vi "Measurement UI.vi"() -> ()   [LabVIEW 2025, in "CAN-LIN Raw Bus Capture UI.lvlib"]
uses:
  CAN-LIN Raw Bus Capture UI.lvlib
  Toggle.ctl
  <vilib>/gRPC/LabVIEW gRPC Library/Shared/grpcId.ctl
  <vilib>/Utility/error.llb/whitespace.ctl
  <vilib>/Utility/error.llb/Trim Whitespace One-Sided.vi
  Get Status.vi
  Flush Table.vi
  Create Buffer.vi
  Destroy Table Buffer.vi
  OOB gRPC Client/OOB gRPC Client.lvlib
  <vilib>/gRPC/LabVIEW gRPC Library/grpc-lvsupport-release.lvlib
  Table_Filtering/Table_Filtering.lvlib
panel:
  in  "Tree Data":string[][](array[string])
  in  "Mapping done?":bool
  in  "Table map":map{string, i32}(c390)
  in  "XNET Sessions map":map{u32, refnum<k21>}(c390)
  in  "Tags map":map{string, bool}(c390)
  out "Valid DBC file?":bool
  out "Signals in DBC":i32
  out "Frames in DBC":i32
  in  "Frames Map":map{u32, refnum<k21>}(c390)
  in  "Signals Map":map{u32, refnum<k21>[]}(c390)
  in  "Tree and Table":enum32{"Trace window", "Signal table"}(tab)
  out "Frames":string(tree)
  out "Signals":string[][](table)
  in  "HELP":bool
  out "IsRestarting?":bool
  out "Table Buffer":i32
  out "Error (Logic)":string
  out "Status Message":string
  in  "SAVE FORMAT":u16(ring) items=["TDMS", "CSV"]
  out "Connection":bool
  in  "Clear Trace":bool
  in  "Bus Type":string="CAN"
  in  "Lin Interface":string
  in  "Can Interface":string
  in  "PauseResume":bool
  in  "Path":path
  in  "Save":bool
  in  "Filter":string
  in  "SortByID":bool
  out "Status":string
  in  "SETTINGS":enum32{"CAN", "LIN"}(tab)
  in  "IO Mode":enum32{"CAN", "CAN FD", "CAN FD + BRS"}(ring)
  in  "FD ISO Mode":enum32{"ISO", "Non ISO", "Legacy ISO"}(ring)
  in  "Baudrate":u32=125000
  in  "FD Baudrate":u32=1000000
  in  "Termination CAN":T1
  in  "INTERFACE NAME CAN":refnum<k21>
  in  "DBC path":path
  in  "Termination LIN":T1
  in  "INTERFACE NAME LIN":refnum<k21>
  out "Buffer Size":i32
  out "OOB gRPC Port":i32
  # "CONFIGURATION"
  # "CONTROL"
  # "DBC INFORMATION"
  # "STATUS"
  # "CAN Settings"
  # "LIN Settings"
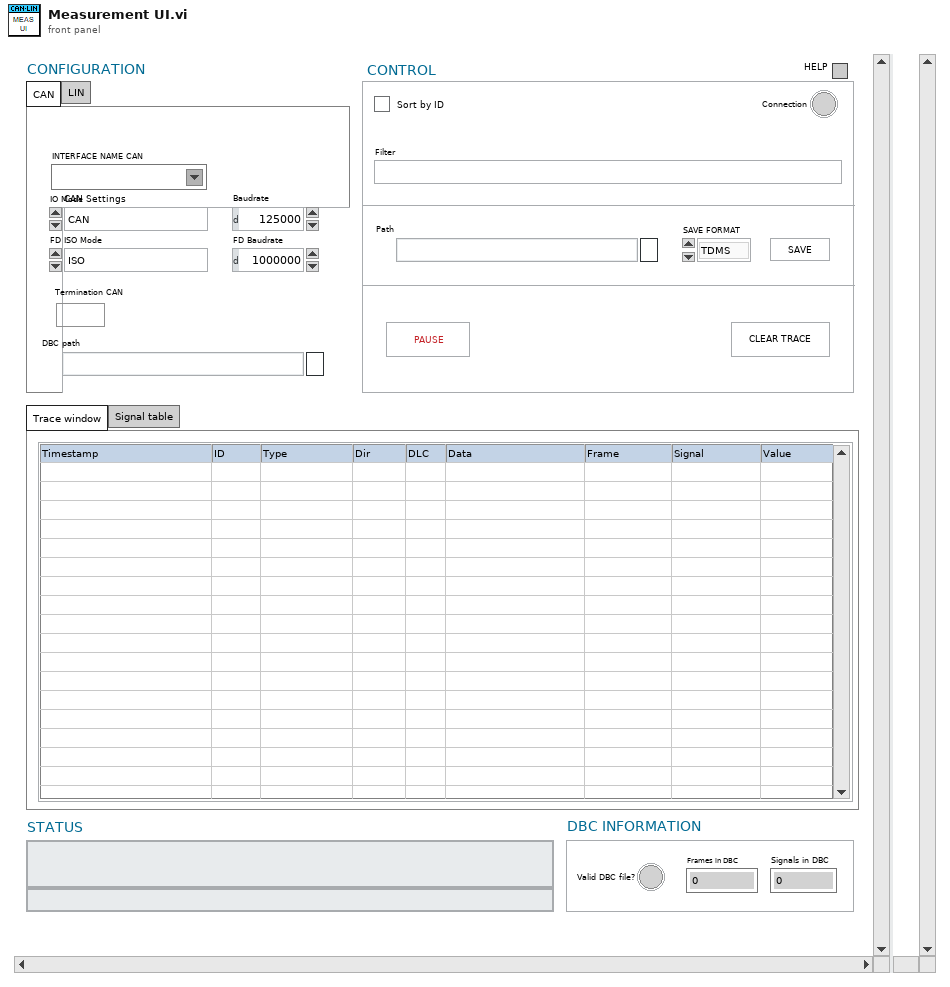
[diagram p1: front panel]
types:
  T1 = typedef "Toggle.ctl" = bool
  T2 = typedef "grpc-lvsupport-release.lvlib/grpcId.ctl" = u64
  T3 = cluster{"Tree Data":refnum<vi>, "Mapping done?":refnum<vi>, "Table map":refnum<vi>, "Tags map":refnum<vi>, "XNET Sessions map":refnum<vi>, "Signals":refnum<vi>, "PauseResume":refnum<vi>, "Clear Trace":refnum<vi>, "Path":refnum<vi>, "SAVE FORMAT":refnum<vi>, "Save":refnum<vi>, "Bus Type":refnum<vi>, "Filter":refnum<vi>, "SortByID":refnum<vi>, "Status Message":refnum<vi>, "Frames":refnum<vi>, "DBC path":refnum<vi>, "Signals Map":refnum<vi>, "Frames Map":refnum<vi>, "Frames in DBC":refnum<vi>, "Signals in DBC":refnum<vi>, "Valid DBC file?":refnum<vi>}
  T4 = typedef "whitespace.ctl" = u16
  T5 = cluster{"FIELD":string, "OPERATOR":string, "VALUE":string}[]
  T6 = enum32{"Page Enabled", "Page Disabled", "Page Disabled & Grayed"}
  T7 = enum8{"Enabled", "Disabled", "Disabled and Grayed Out"}
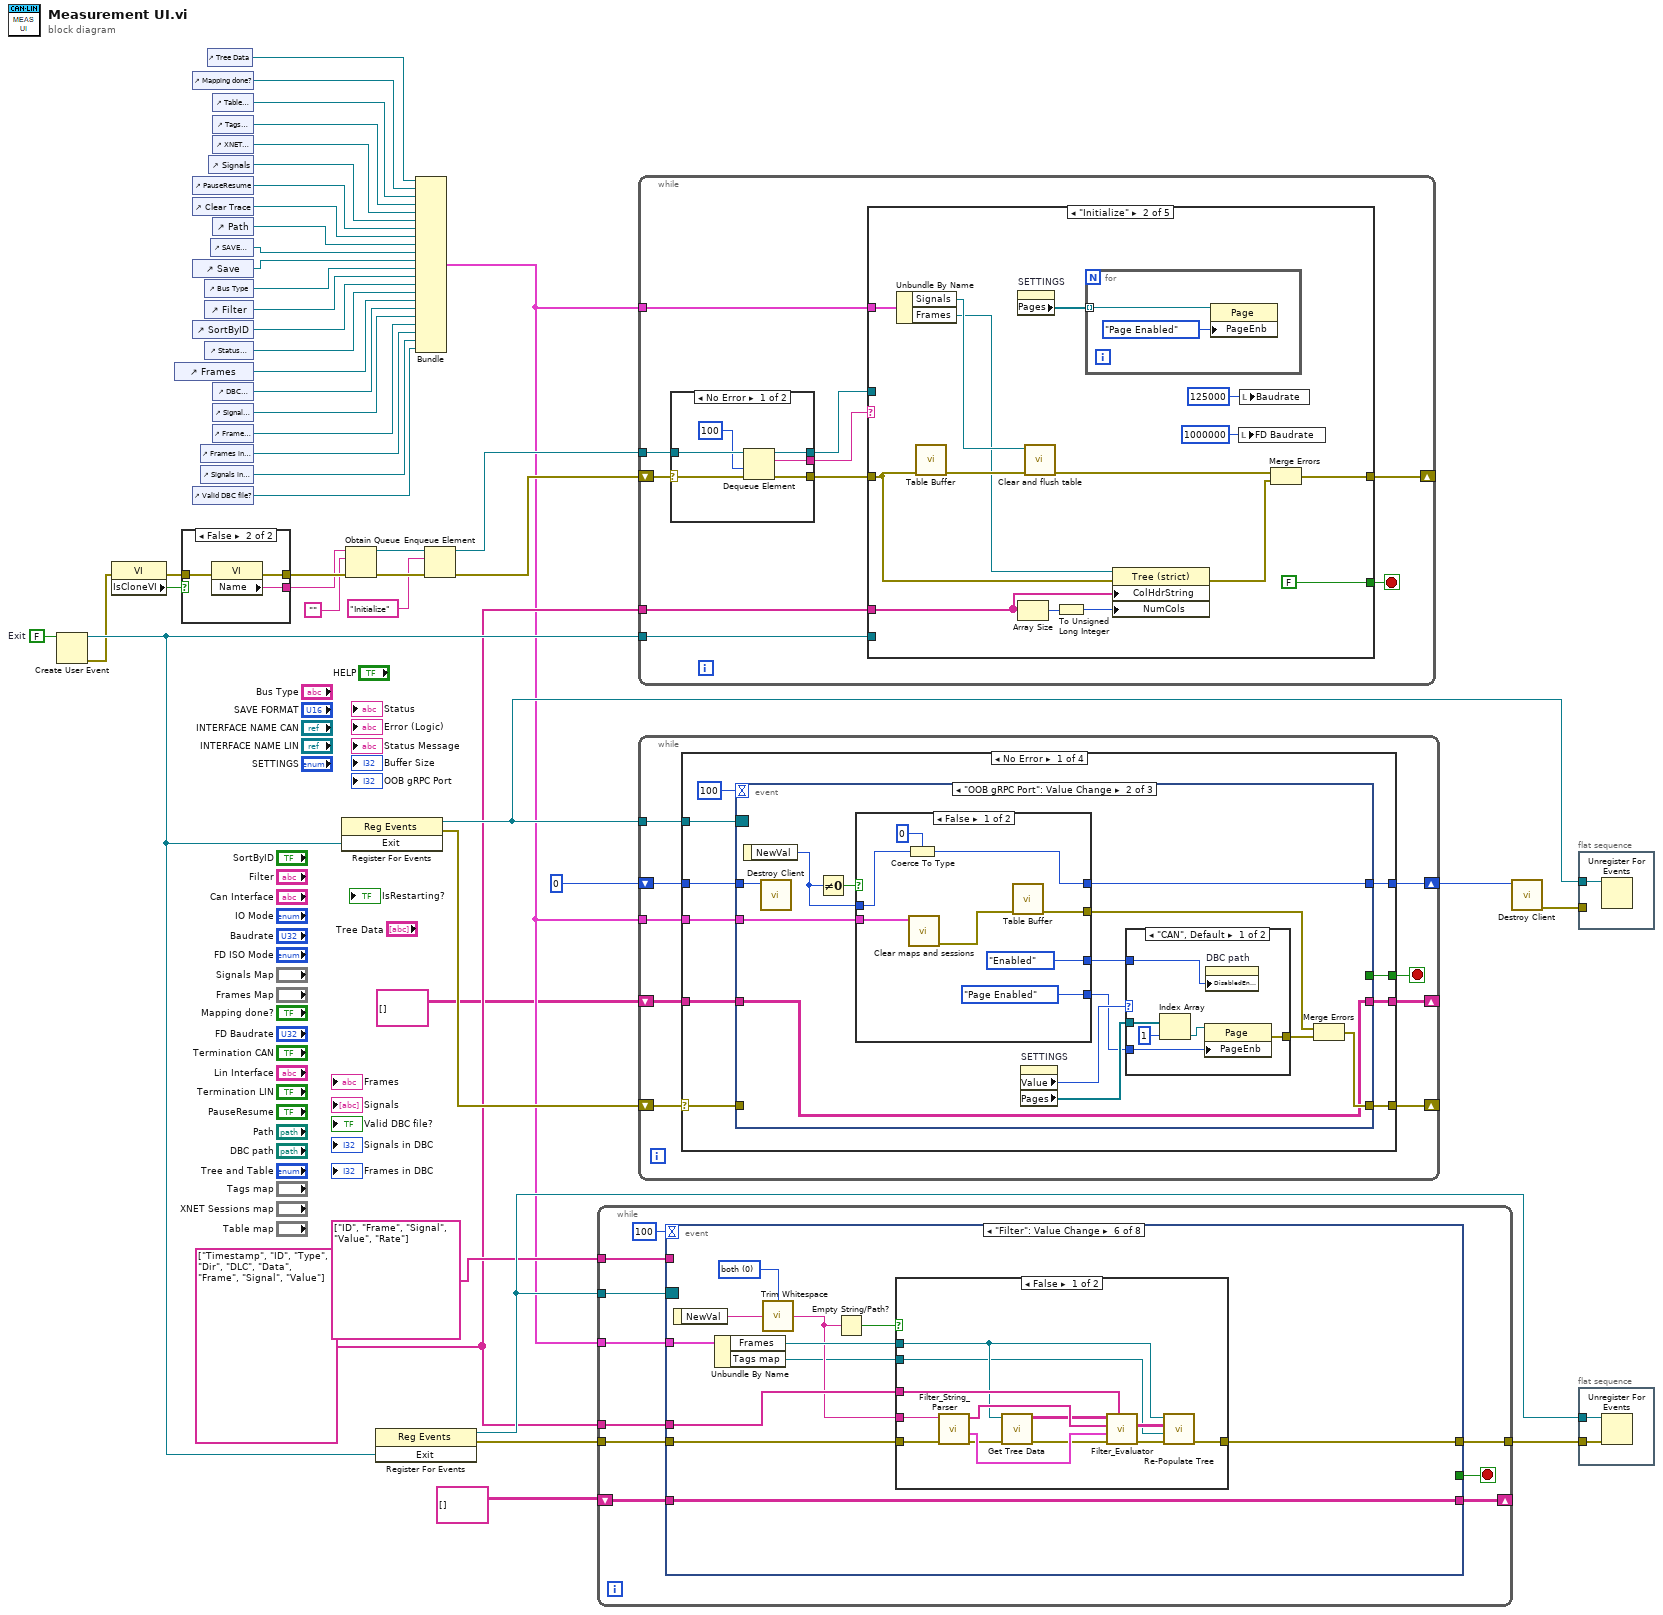
[diagram p0: block diagram]
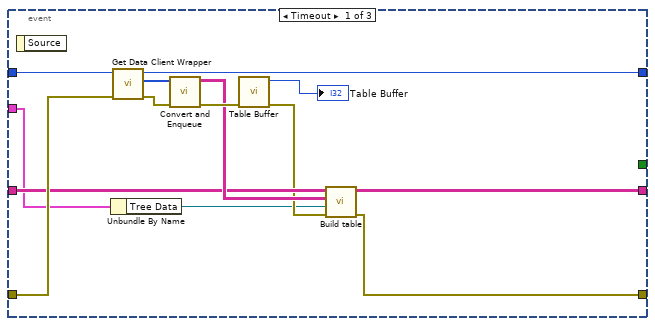
[diagram p2: hidden frame]
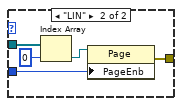
[diagram p3: hidden frame]
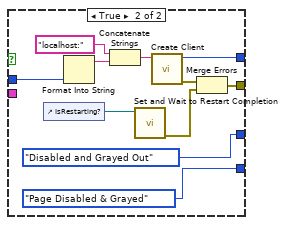
[diagram p4: hidden frame]
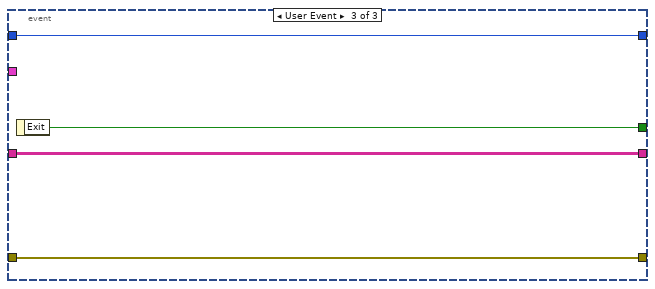
[diagram p5: hidden frame]
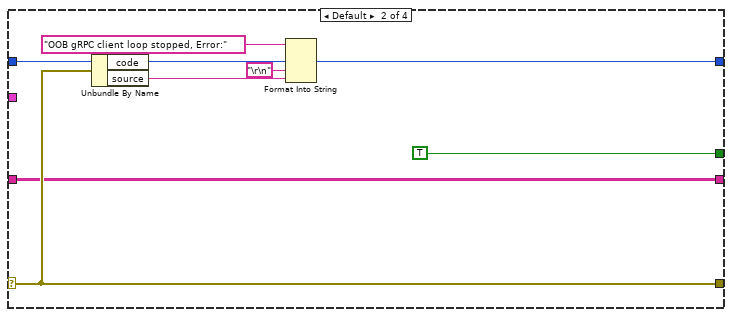
[diagram p6: hidden frame]
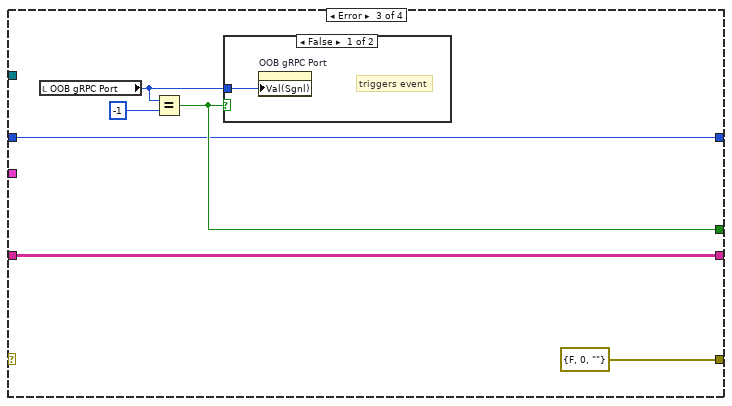
[diagram p7: hidden frame]
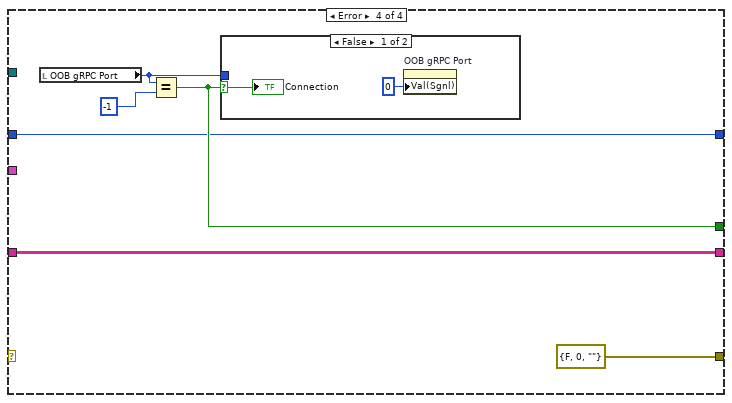
[diagram p9: hidden frame]
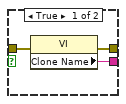
[diagram p11: hidden frame]
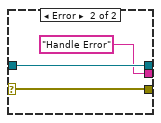
[diagram p12: hidden frame]
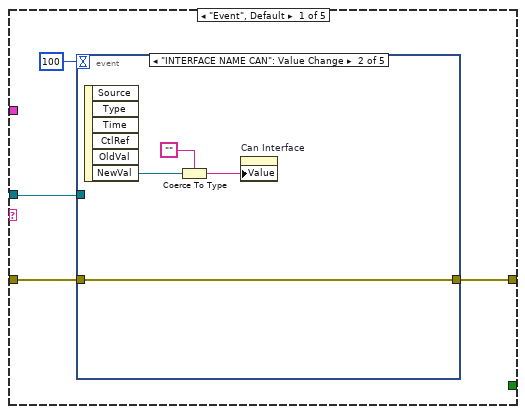
[diagram p13: hidden frame]
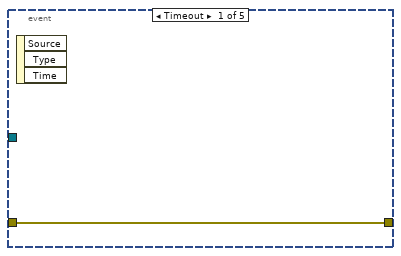
[diagram p14: hidden frame]
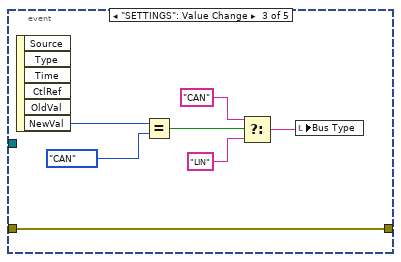
[diagram p15: hidden frame]
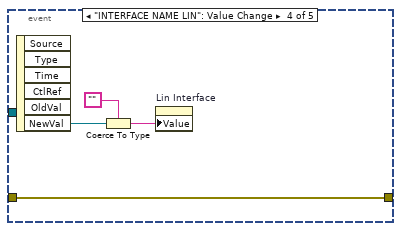
[diagram p16: hidden frame]
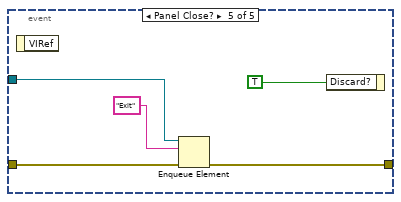
[diagram p17: hidden frame]
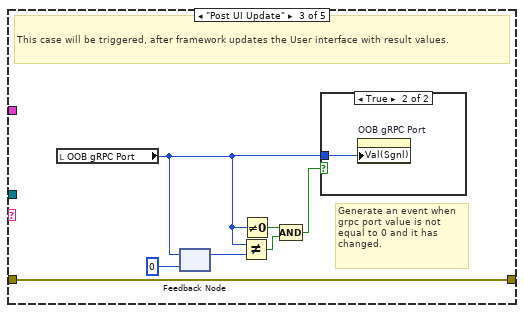
[diagram p18: hidden frame]
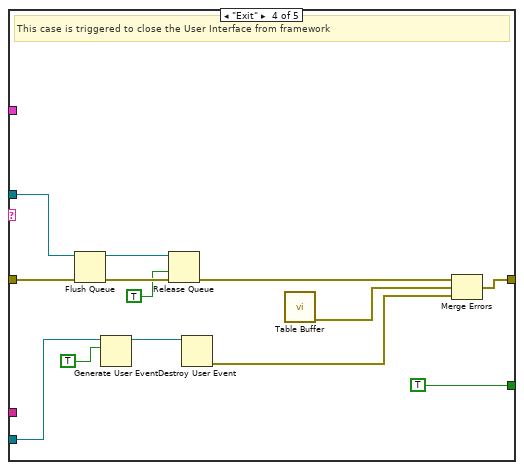
[diagram p20: hidden frame]
diagram:
  w16 = string[] ["Timestamp", "ID", "Type", "Dir", "DLC", "Data", "Frame", "Signal", "Value"] ("Headers")
  w40 = FALSE  # Exit
  n1 = Create User Event(user event datatype=w40) -> (user event=w34:refnum<user-event>, error out=w6:errorcluster)  [unwired: 1 in]
  n2 = property class="VI"(error in=w6) -> (error out=w41:errorcluster, "IsCloneVI"=w42:bool)  [unwired: 1 in, 1 out]
  n3 = control-ref of="Frames"() -> (w20:refnum<vi>)
  n4 = case shown="False" w42 {
    tunnel: [w51 w54] -> w48
    tunnel: [w50 w53] -> w47
    tunnel: w41 -> [w49 w52]
    frame True {
      n5 = property class="VI"(error in=w49) -> (error out=w51:errorcluster, "Clone Name"=w50:string)  [unwired: 1 in, 1 out]
    }
    frame False {
      n6 = property class="VI"(error in=w52) -> (error out=w54:errorcluster, "Name"=w53:string)  [unwired: 1 in, 1 out]
    }
  }
  n7 = control-ref of="Mapping done?"() -> (w4:refnum<vi>)
  n8 = control-ref of="PauseResume"() -> (w24:refnum<vi>)
  n9 = control-ref of="Clear Trace"() -> (w32:refnum<vi>)
  n10 = control-ref of="Save"() -> (w29:refnum<vi>)
  n11 = control-ref of="SortByID"() -> (w27:refnum<vi>)
  n12 = control-ref of="Valid DBC file?"() -> (w12:refnum<vi>)
  n13 = control-ref of="Frames in DBC"() -> (w14:refnum<vi>)
  n14 = control-ref of="Signals in DBC"() -> (w13:refnum<vi>)
  n15 = control-ref of="Bus Type"() -> (w28:refnum<vi>)
  n16 = control-ref of="Filter"() -> (w26:refnum<vi>)
  n17 = control-ref of="Status Message"() -> (w25:refnum<vi>)
  n18 = control-ref of="Tree Data"() -> (w1:refnum<vi>)
  n19 = control-ref of="Signals"() -> (w33:refnum<vi>)
  n20 = control-ref of="SAVE FORMAT"() -> (w30:refnum<vi>)
  n21 = control-ref of="Table map"() -> (w9:refnum<vi>)
  n22 = control-ref of="Tags map"() -> (w11:refnum<vi>)
  n23 = control-ref of="XNET Sessions map"() -> (w10:refnum<vi>)
  n24 = control-ref of="Path"() -> (w31:refnum<vi>)
  n25 = control-ref of="DBC path"() -> (w21:refnum<vi>)
  n26 = control-ref of="Signals Map"() -> (w17:refnum<vi>)
  n27 = control-ref of="Frames Map"() -> (w18:refnum<vi>)
  n28 = register-events(w34) -> (reference out=w36:refnum<event-registration>, error out=w39:errorcluster)  [unwired: 2 in]
  n29 = Obtain Queue(name (unnamed)=w47, element data type="", error in (no error)=w48) -> (queue out=w45:refnum<queue>, error out=w46:errorcluster)  [unwired: 2 in, 1 out]
  n30 = register-events(w34) -> (reference out=w23:refnum<event-registration>, error out=w7:errorcluster)  [unwired: 2 in]
  n31 = Bundle("Tree Data"=w1, "Mapping done?"=w4, "Table map"=w9, "Tags map"=w11, "XNET Sessions map"=w10, "Signals"=w33, "PauseResume"=w24, "Clear Trace"=w32, "Path"=w31, "SAVE FORMAT"=w30, "Save"=w29, "Bus Type"=w28, "Filter"=w26, "SortByID"=w27, "Status Message"=w25, "Frames"=w20, "DBC path"=w21, "Signals Map"=w17, "Frames Map"=w18, "Frames in DBC"=w14, "Signals in DBC"=w13, "Valid DBC file?"=w12) -> (w3:T3)  [unwired: 1 in]
  n32 = Enqueue Element(queue=w45, element="Initialize", error in (no error)=w46) -> (queue out=w15:refnum<queue>, error out=w8:errorcluster)  [unwired: 1 in, 1 out]
  n33 = while {
    tunnel: w7 -> [w64]
    tunnel: [w59] -> w5
    tunnel: w23 -> [w63]
    tunnel: w3 -> [w60]
    shift-right: [w57] -> _
    shift-left: string[][] [] ("Table Data out") -> [w58]
    tunnel: string[] ["ID", "Frame", "Signal", "Value", "Rate"] ("Signal Table Headers") -> [w56]
    tunnel: w16 -> [w55]
    stop <- w62 stop-if-true
    n34 = event shown="[5] \"Filter\": Value Change" {
      selector: w63 -> [_ _ _ _ _ _ _ _]
      dyn-events: _ -> [_ _ _ _ _ _ _ _]
      timeout: 100 -> [_ _ _ _ _ _ _ _]
      tunnel: w64 -> [w82 w94 w113 w130 w154 w165 w186 w188]
      tunnel: [w89 w93 w112 w129 w147 w162 w185 w188] -> w59
      tunnel: [_ _ _ _ _ _ _ w189] -> w62
      tunnel: w60 -> [w80 _ w109 w131 w156 w166 _ _]
      tunnel: w58 -> [w77 w92 w104 w128 w151 w167 w184 w187]
      tunnel: [w91 w92 w105 w128 w151 w167 w184 w187] -> w57
      tunnel: w56 -> [w83 _ _ _ w150 _ _ _]
      tunnel: w55 -> [_ _ _ w126 _ w164 _ _]
      event Timeout {
        n35 = event-data() -> ()  [unwired: 1 in, 1 out]
        n36 = Unbundle By Name(w80) -> ("Signals"=w85:refnum<vi>, "Filter"=w66:refnum<vi>, "SortByID"=w87:refnum<vi>, "Table map"=w78:refnum<vi>, "PauseResume"=w79:refnum<vi>)
        n37 = call "Map the Signals and Frames.vi"("error in"=w82, "References"=w80) -> ("error out"=w81:errorcluster)  [unwired: 9 in]
        n38 = call "PauseResume.vi"("error in"=w81, "PauseResume Ref"=w79) -> ("error out"=w75:errorcluster, "Data"=w84:string[][])  [unwired: 8 in]
        n39 = property class="VI"(error in=w75) -> (error out=w76:errorcluster, "Panel"=w72:refnum<vi>)  [unwired: 1 in, 1 out]
        n40 = property class="Pnl"(reference=w72, error in=w76, "DeferPanUpdts"=TRUE ("Defer Panel Updates")) -> (error out=w74:errorcluster)  [unwired: 1 out]
        n41 = call "Update Trace Tree.vi"("References"=w80, "error in"=w74, "Data IN"=w84) -> ("error out"=w67:errorcluster, "Signals"=w71:string[][])  [unwired: 7 in]
        n42 = call "Update Table.vi"("Table map"=w78, "error in"=w67, "New Data in"=w71, "Table Data in"=w77) -> ("error out"=w68:errorcluster, "Table Data out"=w91:string[][])  [unwired: 6 in]
        n43 = property class="VI"(error in=w68) -> ("Panel"=w69:refnum<vi>)  [unwired: 1 in, 2 out]
        n44 = property class="Pnl"(reference=w69, "DeferPanUpdts"=FALSE ("Defer Panel Updates")) -> (error out=w65:errorcluster)  [unwired: 1 in, 1 out]
        n45 = Empty Array?(array=w71) -> (empty?=w86:bool)
        n46 = call "SortByID.vi"("Headers"=w83, "Trace"=w85, "error in"=w65, "Unsorted Data"=w91, "SortByID"=w87, "Filter"=w66) -> ("error out"=w90:errorcluster, "Table Control"=w88:string[][])  [unwired: 4 in]
        n47 = call "Programatic Scroll.vi"("error in"=w90, "Pause? (F)"=w86, "Table Ref"=w85, "Trace"=w88) -> ("error out"=w89:errorcluster)  [unwired: 7 in]
      }
      event "Clear Trace": Value Change {
        # "Run when restarting or then button is pressed down."
        n48 = event-data() -> ("NewVal"=w95:bool)  [unwired: 1 in]
        n49 = case shown="False" w95 {
          tunnel: w94 -> [w98 w99]
          tunnel: [w96 w99] -> w93
          frame False {
            n50 = property on="IsRestarting?" class="Bool (strict)"(error in=w98, "Val(Sgnl)"=FALSE ("Value (Signaling)")) -> (error out=w96:errorcluster)  [unwired: 1 in, 1 out]
          }
          frame True {
          }
        }
      }
      event "IsRestarting?": Value Change {
        n51 = event-data() -> ("NewVal"=w111:bool)  [unwired: 1 in]
        n52 = Unbundle By Name(w109) -> ("Table map"=w100:refnum<vi>, "Tags map"=w101:refnum<vi>, "Frames"=w102:refnum<vi>, "Status Message"=w106:refnum<vi>, "Signals"=w108:refnum<vi>)
        n53 = Not(x=w111) -> (.not. x?=w110:bool)
        n54 = call "Clear Table.vi"("error in"=w113, "Confirm? (F)"=w110, "Table in"=w108) -> ("error out"=w107:errorcluster, "T button?"=w103:bool)  [unwired: 7 in]
        n55 = case shown="True" w103 {
          tunnel: [w115 w124] -> w112
          tunnel: w107 -> [w115 w122]
          tunnel: w106 -> [_ w121]
          tunnel: [w114 string[][] [] ("Table Data out")] -> w105
          tunnel: w104 -> [w114 _]
          tunnel: w102 -> [_ w118]
          tunnel: w101 -> [_ w117]
          tunnel: w100 -> [_ w116]
          frame False {
          }
          frame True {
            # "Reset Table when necessary"
            n56 = invoke class="Map (strict)" method="Reinit To Default"(reference=w116) -> ()  [unwired: 2 in, 3 out]
            n57 = invoke class="Map (strict)" method="Reinit To Default"(reference=w117) -> ()  [unwired: 2 in, 3 out]
            n58 = property class="Str"(reference=w121, error in=w122, "Value"="") -> (error out=w123:errorcluster)  [unwired: 1 out]
            n59 = property on="IsRestarting?" class="Bool (strict)"(error in=w123, "Value"=FALSE ("IsRestarting?")) -> (error out=w124:errorcluster)  [unwired: 1 in, 1 out]
            n60 = invoke on="Invoke Node" class="Tree (strict)" method="Edit Tree Items.Delete"(reference=w118) -> ()  [unwired: 4 in, 5 out]
          }
        }
      }
      event "Save": Value Change {
        n61 = event-data() -> ("NewVal"=w127:bool)  [unwired: 1 in]
        n62 = case shown="False" w127 {
          tunnel: w131 -> [_ w145]
          tunnel: w130 -> [w132 w141]
          tunnel: [w132 w139] -> w129
          tunnel: w126 -> [_ w137]
          frame True {
          }
          frame False {
            n63 = Unbundle By Name(w145) -> ("DBC path"=w134:refnum<vi>, "Status Message"=w136:refnum<vi>, "Path"=w144:refnum<vi>, "SAVE FORMAT"=w143:refnum<vi>, "Bus Type"=w142:refnum<vi>, "Tree Data"=w133:refnum<vi>, "Frames"=w135:refnum<vi>)
            n64 = call "Save CAN data.vi"("Frames"=w135, "DBC path"=w134, "Tree Data"=w133, "Headers"=w137, "error in"=w141, "Bus Type"=w142, "Format"=w143, "Path"=w144) -> ("error out"=w140:errorcluster, "Status"=w138:string)  [unwired: 2 in]
            n65 = property class="Str"(reference=w136, error in=w140, "Value"=w138) -> (error out=w139:errorcluster)  [unwired: 1 out]
          }
        }
      }
      event "SortByID": Value Change {
        # "This currently only checks the sorting value change,\nmigth need to check the  Filter Value Change too."
        n66 = event-data() -> ()  [unwired: 1 in, 1 out]
        n67 = Unbundle By Name(w156) -> ("Tags map"=w146:refnum<vi>, "Frames"=w149:refnum<vi>, "Signals"=w153:refnum<vi>, "Filter"=w152:refnum<vi>, "SortByID"=w155:refnum<vi>)
        n68 = call "SortByID.vi"("Headers"=w150, "Trace"=w153, "error in"=w154, "Unsorted Data"=w151, "SortByID"=w155, "Filter"=w152) -> ("error out"=w148:errorcluster)  [unwired: 4 in, 1 out]
        n69 = call "Order tree.vi"("Tags map"=w146, "error in"=w148, "TreeControl in"=w149) -> ("error out"=w147:errorcluster)  [unwired: 8 in]
      }
      event "Filter": Value Change {
        w160 = T4 0 items=["both", "start of string", "end of string"] ("location (both)")
        n70 = event-data() -> ("NewVal"=w161:string)  [unwired: 1 in]
        n71 = Unbundle By Name(w166) -> ("Frames"=w163:refnum<vi>, "Tags map"=w157:refnum<vi>)
        n72 = call <vilib>:"Trim Whitespace.vi"("string"=w161, "location (both)"=w160) -> ("trimmed string"=w159:string)
        n73 = Empty String/Path?(string/path=w159) -> (empty?=w158:bool)
        n74 = case shown="False" w158 {
          tunnel: w165 -> [w180 w181]
          tunnel: w164 -> [w177 _]
          tunnel: w163 -> [w171 _]
          tunnel: [w170 w181] -> w162
          tunnel: w159 -> [w169 _]
          tunnel: w157 -> [w168 _]
          frame False {
            n75 = call "Filter_String_Parser.vi"("error in"=w180, "Filter String"=w169) -> ("error constant"=w174:errorcluster, "Comparators"=w179:T5, "Boolean Connectors"=w178:string[])  [unwired: 7 in]
            n76 = call "Get Tree Data.vi"("error in"=w174, "Tree ref"=w171) -> ("error out"=w175:errorcluster, "Array"=w176:string[][])  [unwired: 8 in]
            n77 = call "Filter_Evaluator.vi"("Headers"=w177, "Error"=w175, "Comparators"=w179, "Boolean Connectors"=w178, "Prefiltered Data"=w176) -> ("Error Out"=w172:errorcluster, "Filtered Array"=w173:string[][])  [unwired: 4 in, 1 out]
            n78 = call "Re-Populate Tree.vi"("error in"=w172, "Tags map"=w168, "Data in"=w173, "TreeControl in"=w171) -> ("error out"=w170:errorcluster)  [unwired: 7 in]
          }
          frame True {
          }
        }
      }
      event "HELP": Value Change {
        n79 = event-data() -> ("NewVal"=w183:bool)  [unwired: 1 in]
        n80 = call "Open Help PDF.vi"("error in"=w186, "NewVal"=w183, "Path after documentation"=path "CAN-LIN Raw Bus Capture.pdf") -> ("error out"=w185:errorcluster)  [unwired: 8 in]
      }
      event User Event {
        n81 = event-data() -> ("Exit"=w189:bool)  [unwired: 1 in]
      }
    }
  }
  n82 = while {
    shift-right: [w194] -> _
    shift-left: w8 -> [w199]
    tunnel: w15 -> [w197]
    tunnel: w34 -> [w192]
    tunnel: w3 -> [w191]
    tunnel: w16 -> [w190]
    stop <- w193 stop-if-true
    n83 = case shown="No Error" w199 {
      selector: w199 -> [w205 w208]
      tunnel: [w204 w208] -> w198
      tunnel: w197 -> [w203 w207]
      tunnel: [w202 w207] -> w196
      tunnel: [w201 "Handle Error"] -> w195
      frame No Error {
        n84 = Dequeue Element(queue=w203, timeout in ms (-1)=100, error in (no error)=w205) -> (queue out=w202:refnum<queue>, element=w201:string, error out=w204:errorcluster)  [unwired: 1 out]
      }
      frame Error {
      }
    }
    n85 = case shown="\"Initialize\"" w195 {
      tunnel: w198 -> [w211 w236 w251 w271 w276]
      tunnel: w196 -> [w210 _ _ w269 w275]
      tunnel: [w212 w239 w251 w260 w276] -> w194
      tunnel: [_ FALSE _ TRUE _] -> w193
      tunnel: w192 -> [_ _ _ w263 _]
      tunnel: w191 -> [_ w234 _ _ _]
      tunnel: w190 -> [_ w235 _ _ _]
      frame "Event", Default {
        n86 = event shown="[1] \"INTERFACE NAME CAN\": Value Change" {
          selector: _ -> [_ _ _ _ _]
          dyn-events: _ -> [_ _ _ _ _]
          timeout: 100 -> [_ _ _ _ _]
          tunnel: [w213 w217 w219 w228 w232] -> w212
          tunnel: w211 -> [w213 w217 w219 w228 w233]
          tunnel: w210 -> [_ _ _ _ w231]
          event Timeout {
            n87 = event-data() -> ()  [unwired: 1 in, 3 out]
          }
          event "INTERFACE NAME CAN": Value Change {
            n88 = event-data() -> ("NewVal"=w215:refnum<k21>)  [unwired: 1 in, 5 out]
            n89 = Coerce To Type(0:w215, 1:"") -> (2:w214:string)
            n90 = property on="Can Interface" class="Str"("Value"=w214) -> ()  [unwired: 2 in, 2 out]
          }
          event "SETTINGS": Value Change {
            n91 = event-data() -> ("NewVal"=w224:enum32{"CAN", "LIN"})  [unwired: 1 in, 5 out]
            n92 = Equal?(x=w224, y=enum32{"CAN", "LIN"}."CAN") -> (x = y?=w222:bool)
            n93 = Select(t="CAN", s=w222, f="LIN") -> (s? t:f=w218:string)
            n94 = local write "Bus Type"(w218) -> ()
          }
          event "INTERFACE NAME LIN": Value Change {
            n95 = event-data() -> ("NewVal"=w225:refnum<k21>)  [unwired: 1 in, 5 out]
            n96 = Coerce To Type(0:w225, 1:"") -> (2:w226:string)
            n97 = property on="Lin Interface" class="Str"("Value"=w226) -> ()  [unwired: 2 in, 2 out]
          }
          event Panel Close? {
            n98 = event-data() -> ()  [unwired: 1 in, 1 out]
            n99 = Enqueue Element(queue=w231, element="Exit", error in (no error)=w233) -> (error out=w232:errorcluster)  [unwired: 1 in, 2 out]
            n100 = event-data("Discard?"=TRUE) -> ()  [unwired: 1 in, 1 out]
          }
        }
      }
      frame "Initialize" {
        n101 = Unbundle By Name(w234) -> ("Signals"=w245:refnum<vi>, "Frames"=w240:refnum<vi>)
        n102 = call-poly "Table Buffer.vi"("error in (no error)"=w236) -> ("error out"=w243:errorcluster)  [unwired: 10 in]
        n103 = property on="SETTINGS" class="TabCtl (strict)"() -> ("Pages"=w244:refnum<vi>[])  [unwired: 2 in, 2 out]
        n104 = Array Size(array=w235) -> (size(s)=w241:i32)
        n105 = call "Clear and flush table.vi"("error in"=w243, "Trace"=w245) -> ("error out"=w238:errorcluster)  [unwired: 9 in]
        n106 = To Unsigned Long Integer(number=w241) -> (unsigned 32bit integer=w242:u32)
        n107 = for {
          tunnel: w244 -> [w250] mode=indexing
          n108 = property class="Page"(reference=w250, "PageEnb"=T6."Page Enabled" ("Page Enabled State")) -> ()  [unwired: 1 in, 2 out]
        }
        n109 = property on="Property Node" class="Tree (strict)"(reference=w240, error in=w236, "ColHdrString"=w235, "NumCols"=w242) -> (error out=w237:errorcluster)  [unwired: 1 out]
        n110 = local write "FD Baudrate"(u32 1000000 ("FD Baudrate")) -> ()
        n111 = local write "Baudrate"(u32 125000 ("Baudrate")) -> ()
        n112 = Merge Errors(w238, w237) -> (w239:errorcluster)
      }
      frame "Post UI Update" {
        # "Generate an event when grpc port value is not equal to 0 and it has changed."
        # "This case will be triggered, after framework updates the User interface with result values."
        n113 = local read "OOB gRPC Port"() -> (w254:i32)
        n114 = feedback #1(0 ("OOB gRPC Port")) -> (w253:i32)
        n115 = feedback-in #1(w254) -> ()
        n116 = Not Equal?(x=w254, y=w253) -> (x != y?=w255:bool)
        n117 = Not Equal To 0?(x=w254) -> (x != 0?=w256:bool)
        n118 = Compound Arithmetic op=AND(w256, w255) -> (w252:bool)
        n119 = case shown="True" w252 {
          tunnel: w254 -> [_ w258]
          frame False {
          }
          frame True {
            n120 = property on="OOB gRPC Port" class="DigNum (strict)"("Val(Sgnl)"=w258) -> ()  [unwired: 2 in, 2 out]
          }
        }
      }
      frame "Exit" {
        # "This case is triggered to close the User Interface from framework"
        n121 = Flush Queue(queue=w269, error in (no error)=w271) -> (queue out=w268:refnum<queue>, error out=w267:errorcluster)  [unwired: 1 out]
        n122 = Generate User Event(user event=w263, event data cluster=TRUE ("event data")) -> (user event out=w265:refnum<user-event>)  [unwired: 2 in, 1 out]
        n123 = Release Queue(queue=w268, force destroy? (F)=TRUE, error in (no error)=w267) -> (error out=w259:errorcluster)  [unwired: 2 out]
        n124 = Destroy User Event(user event=w265) -> (error out=w262:errorcluster)  [unwired: 1 in]
        n125 = call-poly "Table Buffer.vi"() -> ("error out"=w261:errorcluster)  [unwired: 11 in]
        n126 = Merge Errors(w259, w261, w262) -> (w260:errorcluster)
      }
      frame "Handle Error" {
        w274 = "UI main loop stopped, Error: %d - %s" ("format string")
        n127 = Unbundle By Name(w276) -> ("code"=w277:i32, "source"=w272:string)
        n128 = case shown="Default" w276 {
          selector: w276 -> [w278 w283]
          tunnel: [w278 w282] -> _
          tunnel: w275 -> [_ w279]
          frame No Error {
          }
          frame Default {
            n129 = call <vilib>:"Clear Errors.vi"("error in (no error)"=w283) -> ("error out"=w281:errorcluster)  [unwired: 5 in, 1 out]
            n130 = Enqueue Element At Opposite End(queue=w279, element="Exit", error in (no error)=w281) -> (error out=w282:errorcluster)  [unwired: 1 in, 2 out]
          }
        }
        n131 = Format Into String(format string=w274, initial string=w274, w277, w272) -> (resulting string=w273:string)  [unwired: 1 in, 1 out]
        n132 = local write "Status Message"(w273) -> ()
      }
    }
  }
  n133 = while {
    tunnel: w36 -> [w289]
    shift-right: [w290] -> _
    shift-left: w39 -> [w292]
    shift-right: [w287] -> w37
    shift-left: T2 0 ("gRPC ID out") -> [w288]
    tunnel: w3 -> [w286]
    shift-right: [w284] -> _
    shift-left: string[][] [] ("Table Data in") -> [w285]
    stop <- w291 stop-if-true
    n134 = case shown="No Error" w292 {
      selector: w292 -> [w300 w365 _ _]
      tunnel: [w297 TRUE w375 w382] -> w291
      tunnel: [w301 w365 errorcluster {"status"=FALSE, "code"=0, "source"=""} ("error IO") errorcluster {"status"=FALSE, "code"=0, "source"=""} ("error IO")] -> w290
      tunnel: w289 -> [w302 _ _ _]
      tunnel: w288 -> [w299 w370 w374 w381]
      tunnel: [w298 w370 w374 w381] -> w287
      tunnel: w286 -> [w295 _ _ _]
      tunnel: w285 -> [w294 w364 w372 w379]
      tunnel: [w293 w364 w372 w379] -> w284
      frame No Error {
        n135 = event shown="[1] \"OOB gRPC Port\": Value Change" {
          selector: w302 -> [_ _ _]
          dyn-events: _ -> [_ _ _]
          timeout: 100 -> [_ _ _]
          tunnel: [w306 w320 w361] -> w301
          tunnel: w300 -> [w310 _ w361]
          tunnel: w299 -> [w311 w329 w362]
          tunnel: [w316 w328 w362] -> w298
          tunnel: [_ _ w363] -> w297
          tunnel: w295 -> [w304 w318 _]
          tunnel: w294 -> [w308 w317 w360]
          tunnel: [w305 w317 w360] -> w293
          event Timeout {
            n136 = event-data() -> ()  [unwired: 1 in, 1 out]
            n137 = Unbundle By Name(w304) -> ("Tree Data"=w303:refnum<vi>)
            n138 = call "Get Data Client Wrapper.vi"("error in"=w310, "gRPC ID in"=w311) -> ("error out"=w315:errorcluster, "Payload"=w314:u8[], "gRPC ID out"=w316:T2)  [unwired: 7 in]
            n139 = call "Convert and Enqueue.vi"("error in"=w315, "Data"=w314) -> ("error out"=w313:errorcluster, "Table Data"=w309:string[][])  [unwired: 8 in]
            n140 = call-poly "Table Buffer.vi"("error in"=w313) -> ("error out"=w307:errorcluster, "Messages"=→"Table Buffer":i32)  [unwired: 9 in]
            n141 = call "Build table.vi"("error in"=w307, "Tree Data"=w303, "New Data in"=w309, "Tree Data in"=w308) -> ("error out"=w306:errorcluster, "Tree Data out"=w305:string[][])  [unwired: 6 in]
          }
          event "OOB gRPC Port": Value Change {
            n142 = event-data() -> ("NewVal"=w326:i32)  [unwired: 1 in]
            n143 = call "Destroy Client.vi"("gRPC ID"=w329) -> ()  [unwired: 10 in, 1 out]
            n144 = Not Equal To 0?(x=w326) -> (x != 0?=w327:bool)
            n145 = case shown="False" w327 {
              tunnel: [w344 w352] -> w321
              tunnel: w326 -> [w347 w356]
              tunnel: [w345 w355] -> w328
              tunnel: [T6."Page Enabled" ("Page Enabled State") T6."Page Disabled & Grayed" ("Page Enabled State")] -> w323
              tunnel: [T7."Enabled" ("DisabledEnum") T7."Disabled and Grayed Out" ("DisabledEnum")] -> w319
              tunnel: w318 -> [w342 _]
              frame False {
                n146 = Coerce To Type(0:w347, 1:T2 0 ("gRPC ID Out")) -> (2:w345:T2)
                n147 = call "Clear maps and sessions.vi"("References"=w342) -> ("error out"=w341:errorcluster)  [unwired: 10 in]
                n148 = call-poly "Table Buffer.vi"("error in"=w341) -> ("error out"=w344:errorcluster)  [unwired: 10 in]
              }
              frame True {
                n149 = control-ref of="IsRestarting?"() -> (w350:refnum<vi>)
                n150 = Format Into String(w356) -> (resulting string=w359:string)  [unwired: 3 in, 1 out]
                n151 = Concatenate Strings("localhost:" ("string"), w359) -> (w357:string)
                n152 = call "Set and Wait to Restart Completion.vi"("Bool Ref"=w350) -> ("error out"=w351:errorcluster)  [unwired: 10 in]
                n153 = call "Create Client.vi"("address"=w357) -> ("error out"=w353:errorcluster, "gRPC ID Out"=w355:T2)  [unwired: 9 in]
                n154 = Merge Errors(w353, w351) -> (w352:errorcluster)
              }
            }
            n155 = property on="SETTINGS" class="TabCtl (strict)"() -> ("Value"=w325:enum32{"CAN", "LIN"}, "Pages"=w324:refnum<vi>[])  [unwired: 2 in, 2 out]
            n156 = case shown="\"CAN\", Default" w325 {
              tunnel: w324 -> [w335 w340]
              tunnel: w323 -> [w332 w338]
              tunnel: [w331 w336] -> w322
              tunnel: w319 -> [w330 _]
              frame "CAN", Default {
                n157 = Index Array(array=w335, index=1) -> (element=w333:refnum<vi>)
                n158 = property class="Page"(reference=w333, "PageEnb"=w332) -> (error out=w331:errorcluster)  [unwired: 1 in, 1 out]
                n159 = property on="DBC path" class="Path"("DisabledEnum"=w330) -> ()  [unwired: 2 in, 2 out]
              }
              frame "LIN" {
                n160 = Index Array(array=w340, index=0) -> (element=w339:refnum<vi>)
                n161 = property class="Page"(reference=w339, "PageEnb"=w338) -> (error out=w336:errorcluster)  [unwired: 1 in, 1 out]
              }
            }
            n162 = Merge Errors(w321, w322) -> (w320:errorcluster)
          }
          event User Event {
            n163 = event-data() -> ("Exit"=w363:bool)  [unwired: 1 in]
          }
        }
      }
      frame Default {
        n164 = Unbundle By Name(w365) -> ("code"=w369:i32, "source"=w368:string)
        n165 = Format Into String(initial string="OOB gRPC client loop stopped, Error:" ("format string"), w369, "\r\n", w368) -> ()  [unwired: 2 in, 2 out]
      }
      frame Error {
        n166 = local read "OOB gRPC Port"() -> (w377:i32)
        n167 = Equal?(x=w377, y=-1 ("x")) -> (x = y?=w375:bool)
        n168 = case shown="False" w375 {
          tunnel: w377 -> [w378 _]
          frame False {
            # "triggers event"
            n169 = property on="OOB gRPC Port" class="DigNum (strict)"("Val(Sgnl)"=w378) -> ()  [unwired: 2 in, 2 out]
          }
          frame True {
          }
        }
      }
      frame Error {
        n170 = local read "OOB gRPC Port"() -> (w384:i32)
        n171 = Equal?(x=w384, y=-1 ("x")) -> (x = y?=w382:bool)
        n172 = case shown="False" w382 {
          selector: w382 -> [w385 _]
          tunnel: w384 -> [_ _]
          frame False {
            n173 = property on="OOB gRPC Port" class="DigNum (strict)"("Val(Sgnl)"=0 ("Value (Signaling)")) -> ()  [unwired: 2 in, 2 out]
            "Connection" <- w385
          }
          frame True {
          }
        }
      }
    }
  }
  n174 = call "Destroy Client.vi"("gRPC ID"=w37) -> ("error out"=w38:errorcluster)  [unwired: 10 in]
  n175 = flat-sequence {
    tunnel: w36 -> [w387]
    tunnel: w38 -> [_]
    frame #0 {
      n176 = Unregister For Events(event registration refnum=w387) -> ()  [unwired: 1 in, 1 out]
    }
  }
  n177 = flat-sequence {
    tunnel: w23 -> [w389]
    tunnel: w5 -> [w388]
    frame #0 {
      n178 = Unregister For Events(event registration refnum=w389, error in=w388) -> ()  [unwired: 1 out]
    }
  }
